vi "Car Wash.vi"() -> ()   [LabVIEW 2013]
doc: "This VI is a automated car wash simulation.\nIn initialize state all the controls will get enable and you have to select the control.\nOn pressing start, Car Warh Indicator start responding according to wash option.\n\nEach LED will glow for 5 sec.\nAfter then it will go to the next LED which is turned on from the wash option input\n\nIf the car position slider's position and wash option are not same then indicator will show Vehicle out of position.\n\nStop Program will stop the VI"
uses:
  Controls/Car Wash Indicators.ctl
  Controls/Wash Options.ctl
  Controls/States.ctl
  Controls/Wash option states.ctl
panel:
  in  "Start":bool
  out "Elapsed Time":dbl format="%0.2f"
  in  "stop":bool
  out "Wash Entry":bool
  in  "Wash Options":T1
  in  "Car Position Slider":u8(slide) max=3 scale=0.0..4.0
  out "Car Wash Indicators":T2
  # "Entry Console"
  # "Car Wash Display"
  # "Car Position Simulation"
  # "Pre-Soak\nH-P Wash\nL-P Wax\nSpot Free Rinse"
  # "Underbody Wash\nBug Remover"
  # "Tire Shine\nAir Dry"
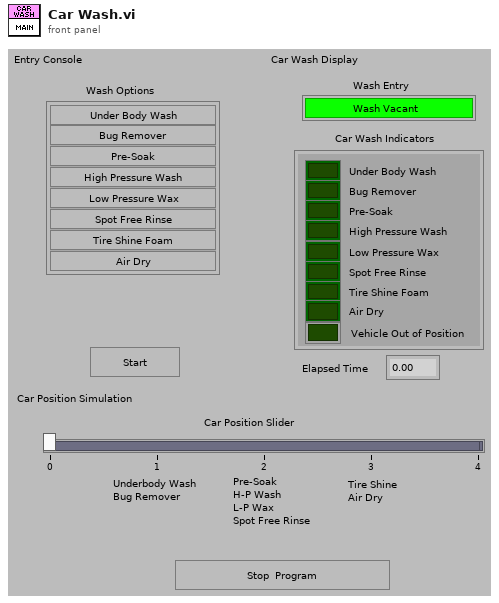
[diagram p1: front panel]
types:
  T1 = typedef "Wash Options.ctl" = cluster{"Underbody Wash":bool, "Bug Remover":bool, "Pre-Soak":bool, "High Pressure Wash":bool, "Low Pressure Wax":bool, "Spot Free Rinse":bool, "Tire Shine Foam":bool, "Air Dry":bool}
  T2 = typedef "Car Wash Indicators.ctl" = cluster{"Under Body Wash":bool, "Bug Remover":bool, "Pre-Soak":bool, "High Pressure Wash":bool, "Low Pressure Wax":bool, "Spot Free Rinse":bool, "Tire Shine Foam":bool, "Air Dry":bool, "Vehicle Out of Position":bool}
  T3 = typedef "Wash option states.ctl" = enum16{"Under Body Wash", "Bug Remover", "Pre-Soak", "HIgh Pressure Wash", "Low Pessure Wax", "Spot Free rinse", "Tire Shine Foam", "Air Dry", "Exit", "Reset "}
  T4 = typedef "States.ctl" = enum16{"Initialize", "Start", "Stop"}
  T5 = enum8{"Enabled", "Disabled", "Disabled and Grayed Out"}
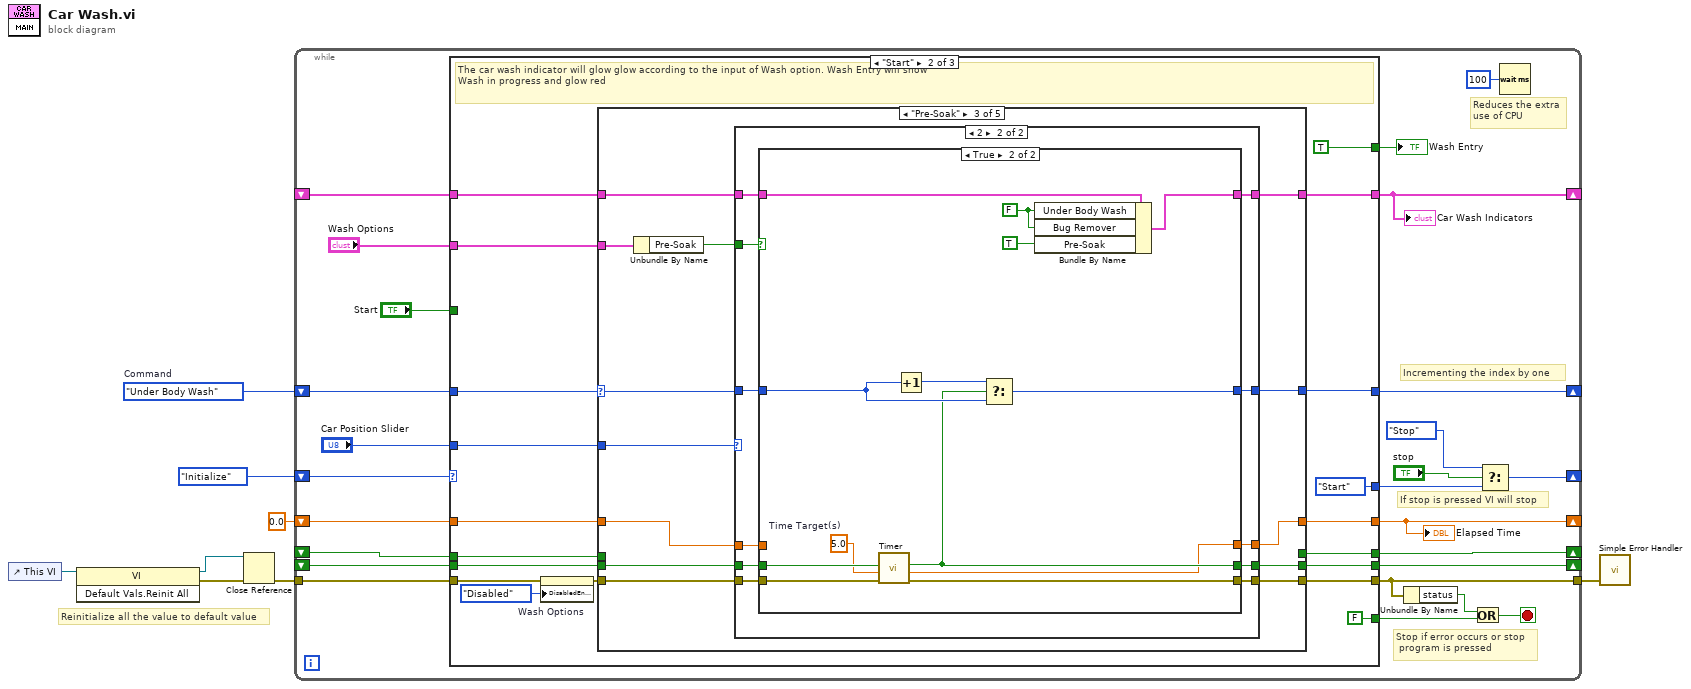
[diagram p0: block diagram]
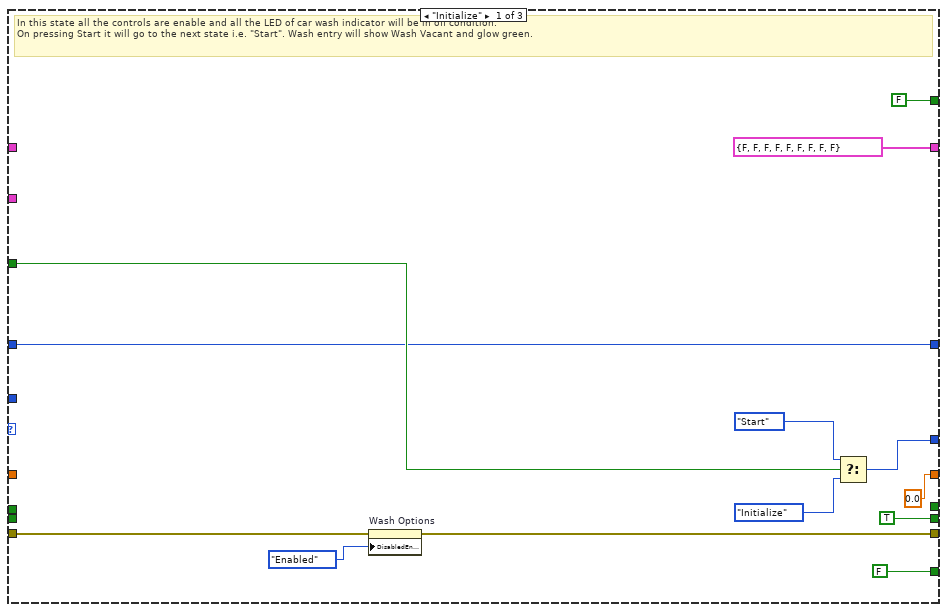
[diagram p2: hidden frame]
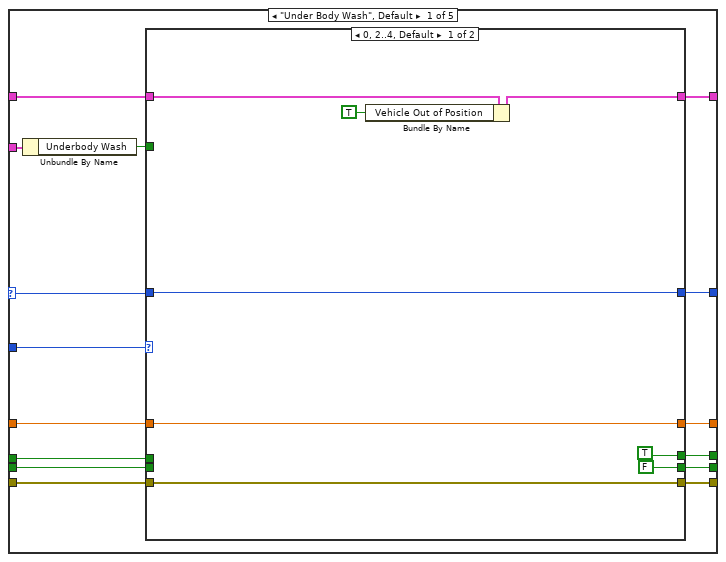
[diagram p3: hidden frame]
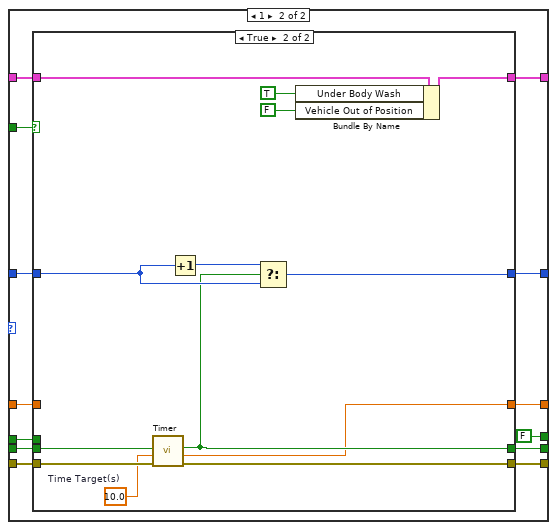
[diagram p4: hidden frame]
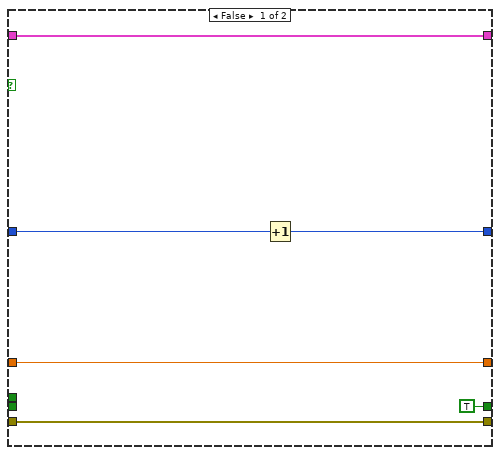
[diagram p5: hidden frame]
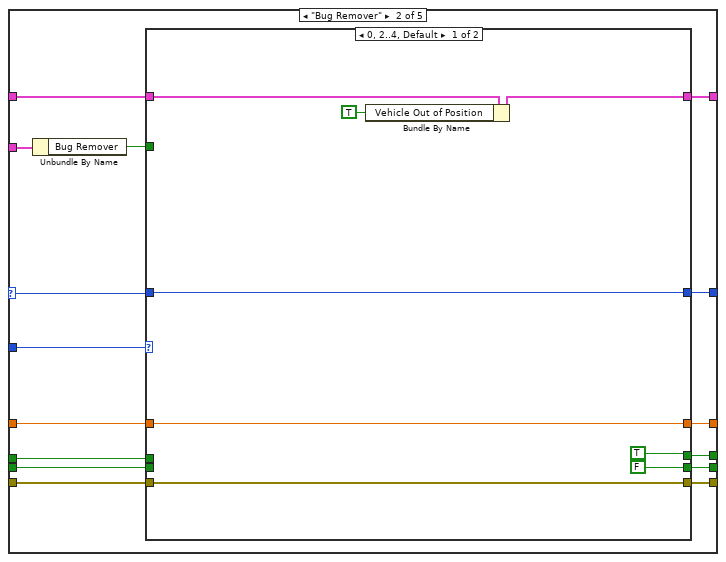
[diagram p6: hidden frame]
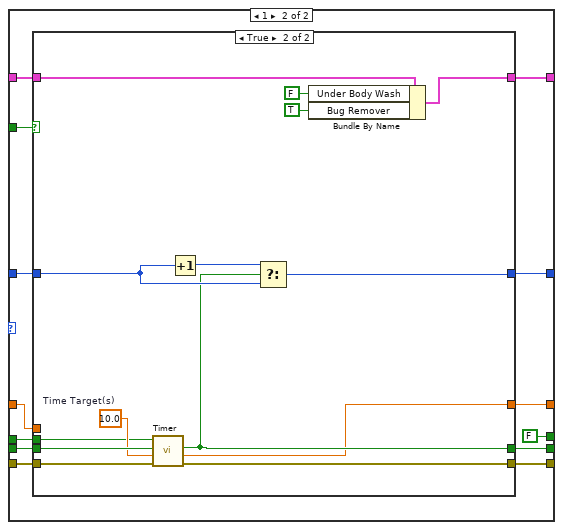
[diagram p7: hidden frame]
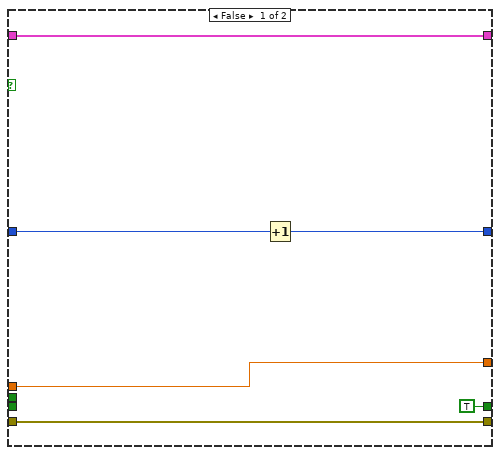
[diagram p8: hidden frame]
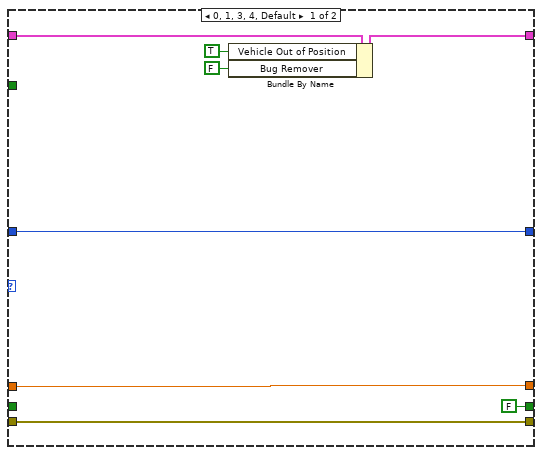
[diagram p9: hidden frame]
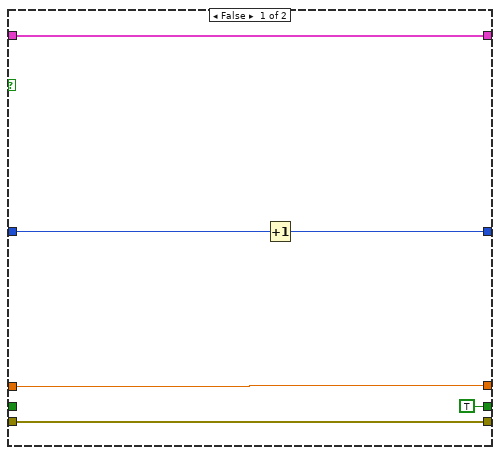
[diagram p10: hidden frame]
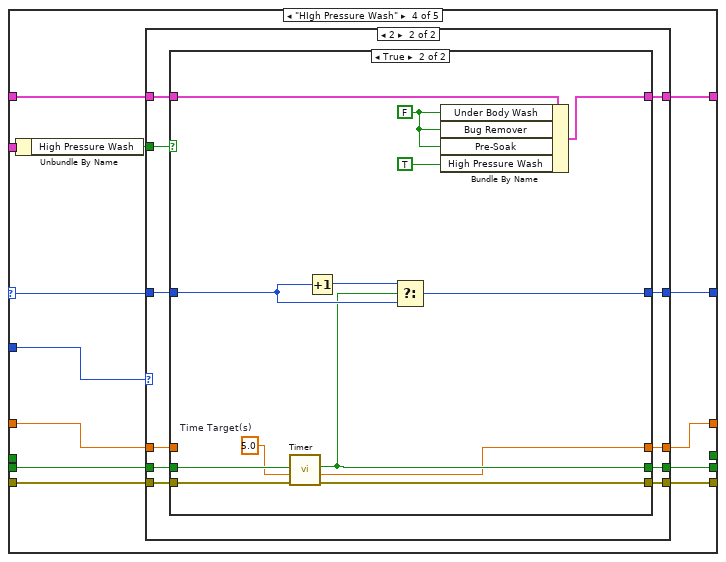
[diagram p11: hidden frame]
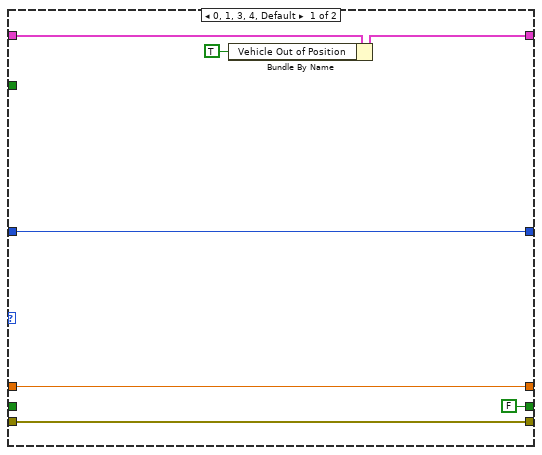
[diagram p12: hidden frame]
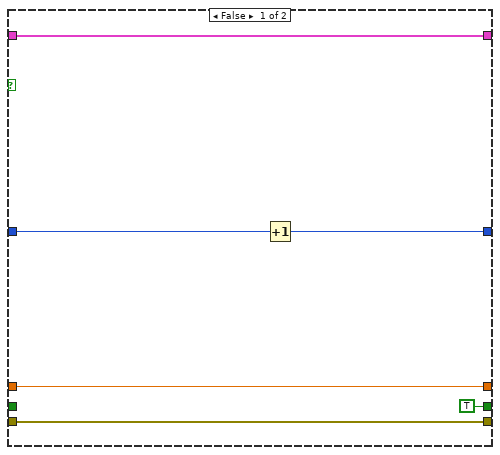
[diagram p13: hidden frame]
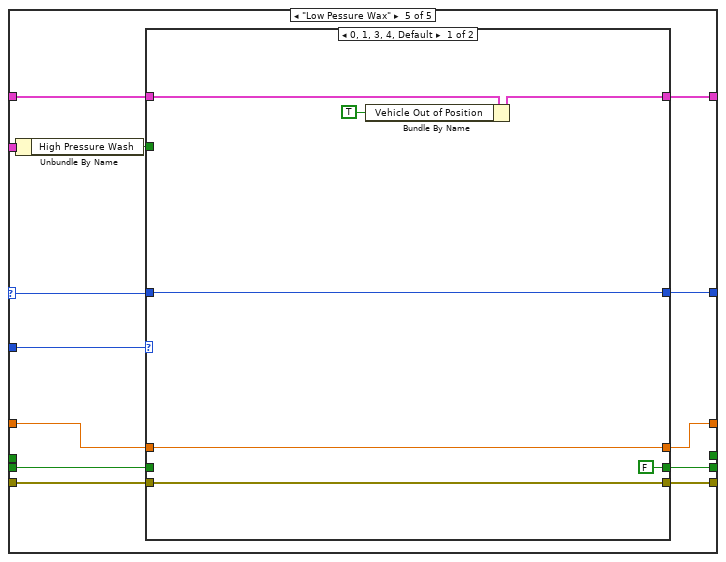
[diagram p14: hidden frame]
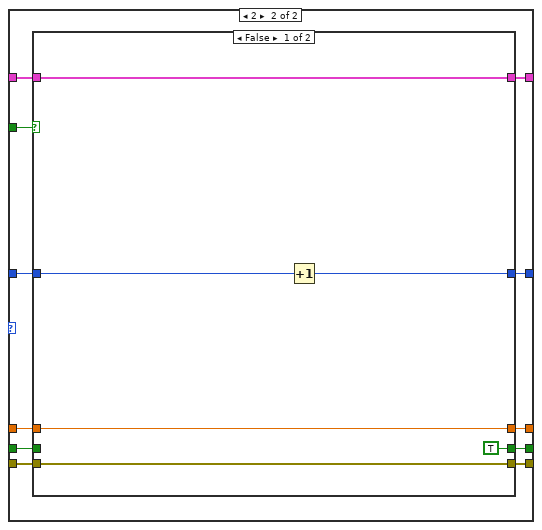
[diagram p15: hidden frame]
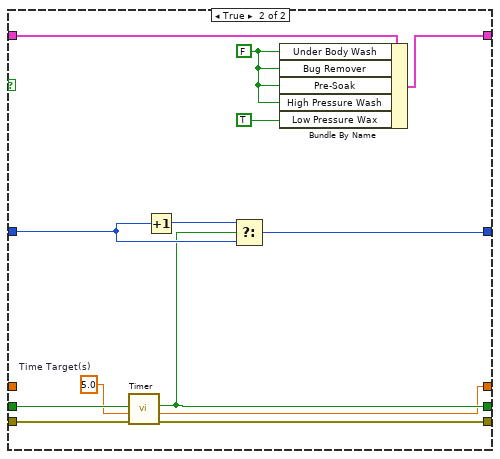
[diagram p16: hidden frame]
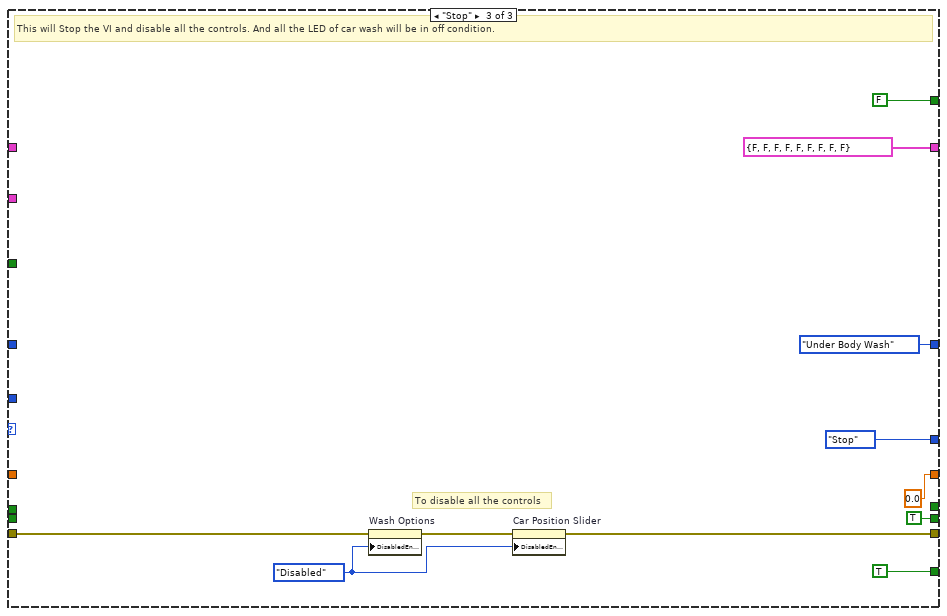
[diagram p17: hidden frame]
diagram:
  w2 = Wash_option_states."Under Body Wash"  # Command
  # "Reinitialize all the value to default value"
  n1 = control-ref of="This VI"() -> (w8:refnum<vi>)
  n2 = invoke class="VI" method="Default Vals.Reinit All"(reference=w8) -> (reference out=w6:refnum<vi>, error out=w7:errorcluster)  [unwired: 2 in, 1 out]
  n3 = Close Reference(reference=w6, error in (no error)=w7) -> (error out=w5:errorcluster)
  n4 = while {
    tunnel: w5 -> [w33]
    tunnel: [w32] -> w4
    shift-right: [w23] -> _
    shift-left: States."Initialize" -> [w28]
    shift-right: [w19] -> _
    shift-left: w2 -> [w20]
    shift-right: [w18] -> _
    shift-left: _ -> [w17]
    shift-right: [w15] -> _
    shift-left: _ -> [w14]
    shift-right: [w12] -> _
    shift-left: 0.0 ("Elapsed TIme") -> [w11]
    shift-right: [w9] -> _
    shift-left: _ -> [w10]
    stop <- w31 stop-if-true
    # "Incrementing the index by one"
    # "Reduces the extra\nuse of CPU"
    # "If stop is pressed VI will stop"
    # "Stop if error occurs or stop\n program is pressed"
    n5 = case shown="\"Start\"" w28 {
      tunnel: w33 -> [w44 w62 w336]
      tunnel: [w38 w56 w331] -> w32
      tunnel: [FALSE FALSE TRUE] -> w29
      tunnel: [FALSE TRUE FALSE] -> w27
      tunnel: [w41 States."Start" States."Stop"] -> w24
      tunnel: [T2 {"Under Body Wash"=FALSE, "Bug Remover"=FALSE, "Pre-Soak"=FALSE, "High Pressure Wash"=FALSE, "Low Pressure Wax"=FALSE, "Spot Free Rinse"=FALSE, "Tire Shine Foam"=FALSE, "Air Dry"=FALSE, "Vehicle Out of Position"=FALSE} ("Car Wash Indicators") w59 T2 {"Under Body Wash"=FALSE, "Bug Remover"=FALSE, "Pre-Soak"=FALSE, "High Pressure Wash"=FALSE, "Low Pressure Wax"=FALSE, "Spot Free Rinse"=FALSE, "Tire Shine Foam"=FALSE, "Air Dry"=FALSE, "Vehicle Out of Position"=FALSE} ("Car Wash Indicators")] -> w15
      tunnel: "Wash Options" -> [_ w52 _]
      tunnel: w20 -> [w35 w58 _]
      tunnel: [w35 w54 Wash_option_states."Under Body Wash" ("Command")] -> w19
      tunnel: [TRUE w51 TRUE] -> w18
      tunnel: w17 -> [_ w53 _]
      tunnel: "Start" -> [w36 _ _]
      tunnel: w14 -> [_ w60 _]
      tunnel: "Car Position Slider" -> [_ w55 _]
      tunnel: [0.0 ("Elapsed TIme") w50 0.0 ("Elapsed TIme")] -> w12
      tunnel: w11 -> [_ w49 _]
      tunnel: w10 -> [_ w48 _]
      tunnel: [_ w47 _] -> w9
      frame "Initialize" {
        # "In this state all the controls are enable and all the LED of car wash indicator will be in off condition.\nOn pressing Start it will go to the next state i.e. \"Start\". Wash entry will show Wash Vacant and glow green."
        n6 = property on="Wash Options" class="Clust (strict)"(error in=w44, "DisabledEnum"=T5."Enabled" ("Disabled")) -> (error out=w38:errorcluster)  [unwired: 1 in, 1 out]
        n7 = Select(t=States."Start", s=w36, f=States."Initialize") -> (s? t:f=w41:T4)
      }
      frame "Start" {
        # "The car wash indicator will glow glow according to the input of Wash option. Wash Entry will show \nWash in progress and glow red"
        n8 = property on="Wash Options" class="Clust (strict)"(error in=w62, "DisabledEnum"=T5."Disabled" ("Disabled")) -> (error out=w57:errorcluster)  [unwired: 1 in, 1 out]
        n9 = case shown="\"Pre-Soak\"" w58 {
          selector: w58 -> [w75 w130 w184 w235 w285]
          tunnel: w60 -> [w76 w131 w185 w236 w286]
          tunnel: [w77 w132 w186 w237 w287] -> w59
          tunnel: w57 -> [w80 w135 w189 w240 w290]
          tunnel: [w79 w134 w188 w239 w289] -> w56
          tunnel: w55 -> [w78 w133 w187 w238 w288]
          tunnel: [w74 w129 w183 w234 w284] -> w54
          tunnel: w53 -> [w73 w128 w182 w233 w283]
          tunnel: w52 -> [w72 w127 w181 w232 w282]
          tunnel: [w70 w125 w179 w230 w280] -> w51
          tunnel: [w69 w124 w178 w229 w279] -> w50
          tunnel: w49 -> [w68 w123 w177 w228 w278]
          tunnel: w48 -> [w67 w121 _ _ _]
          tunnel: [w66 w122 _ _ _] -> w47
          frame "Under Body Wash", Default {
            n10 = Unbundle By Name(w72) -> ("Underbody Wash"=w71:bool)
            n11 = case shown="0, 2..4, Default" w78 {
              tunnel: w80 -> [w83 w101]
              tunnel: [w83 w100] -> w79
              tunnel: [w87 w99] -> w77
              tunnel: w76 -> [w88 w98]
              tunnel: w75 -> [w85 w97]
              tunnel: [w85 w96] -> w74
              tunnel: w73 -> [_ w95]
              tunnel: w71 -> [_ w94]
              tunnel: [FALSE ("Elapsed?") w93] -> w70
              tunnel: [w81 w91] -> w69
              tunnel: w68 -> [w81 w92]
              tunnel: w67 -> [_ w90]
              tunnel: [TRUE ("Elapsed?") FALSE ("Elapsed?")] -> w66
              frame 0, 2..4, Default {
                n12 = Bundle By Name(cluster=w88, "Vehicle Out of Position"=TRUE) -> (w87:T2)
              }
              frame 1 {
                n13 = case shown="True" w94 {
                  tunnel: w101 -> [w104 w117]
                  tunnel: [w104 w116] -> w100
                  tunnel: [w106 w119] -> w99
                  tunnel: w98 -> [w106 w120]
                  tunnel: w97 -> [w107 w113]
                  tunnel: [w105 w114] -> w96
                  tunnel: w95 -> [_ w115]
                  tunnel: [TRUE ("Elapsed?") w111] -> w93
                  tunnel: w92 -> [w102 _]
                  tunnel: [w102 w109] -> w91
                  tunnel: w90 -> [_ _]
                  frame False {
                    n14 = Increment(x=w107) -> (x+1=w105:T3)
                  }
                  frame True {
                    w110 = 10.0  # Time Target(s)
                    n15 = call "Timer.vi"("error in (no error)"=w117, "Time Target(s)"=w110, "Reset"=w115) -> ("error out"=w116:errorcluster, "Elapsed TIme"=w109:dbl, "Elapsed?"=w111:bool)  [unwired: 6 in]
                    n16 = Increment(x=w113) -> (x+1=w112:T3)
                    n17 = Select(t=w112, s=w111, f=w113) -> (s? t:f=w114:T3)
                    n18 = Bundle By Name(cluster=w120, "Under Body Wash"=TRUE, "Vehicle Out of Position"=FALSE) -> (w119:T2)
                  }
                }
              }
            }
          }
          frame "Bug Remover" {
            n19 = Unbundle By Name(w127) -> ("Bug Remover"=w126:bool)
            n20 = case shown="0, 2..4, Default" w133 {
              tunnel: w135 -> [w138 w156]
              tunnel: [w138 w155] -> w134
              tunnel: [w142 w154] -> w132
              tunnel: w131 -> [w143 w153]
              tunnel: w130 -> [w140 w152]
              tunnel: [w140 w151] -> w129
              tunnel: w128 -> [_ w150]
              tunnel: w126 -> [_ w149]
              tunnel: [FALSE ("Elapsed?") w148] -> w125
              tunnel: [w137 w147] -> w124
              tunnel: w123 -> [w137 w146]
              tunnel: [TRUE ("Elapsed?") FALSE ("Elapsed?")] -> w122
              tunnel: w121 -> [_ w144]
              frame 0, 2..4, Default {
                n21 = Bundle By Name(cluster=w143, "Vehicle Out of Position"=TRUE) -> (w142:T2)
              }
              frame 1 {
                n22 = case shown="True" w149 {
                  tunnel: w156 -> [w159 w173]
                  tunnel: [w159 w172] -> w155
                  tunnel: [w161 w175] -> w154
                  tunnel: w153 -> [w161 w176]
                  tunnel: w152 -> [w162 w169]
                  tunnel: [w160 w170] -> w151
                  tunnel: w150 -> [_ w171]
                  tunnel: [TRUE ("Elapsed?") w167] -> w148
                  tunnel: [w157 w164] -> w147
                  tunnel: w146 -> [w157 _]
                  tunnel: w144 -> [_ w163]
                  frame False {
                    n23 = Increment(x=w162) -> (x+1=w160:T3)
                  }
                  frame True {
                    w166 = 10.0  # Time Target(s)
                    n24 = call "Timer.vi"("error in (no error)"=w173, "Time Target(s)"=w166, "Reset"=w171, "Pause"=w163) -> ("error out"=w172:errorcluster, "Elapsed TIme"=w164:dbl, "Elapsed?"=w167:bool)  [unwired: 5 in]
                    n25 = Increment(x=w169) -> (x+1=w168:T3)
                    n26 = Select(t=w168, s=w167, f=w169) -> (s? t:f=w170:T3)
                    n27 = Bundle By Name(cluster=w176, "Under Body Wash"=FALSE, "Bug Remover"=TRUE) -> (w175:T2)
                  }
                }
              }
            }
          }
          frame "Pre-Soak" {
            n28 = Unbundle By Name(w181) -> ("Pre-Soak"=w180:bool)
            n29 = case shown="2" w187 {
              tunnel: w189 -> [w192 w208]
              tunnel: [w192 w207] -> w188
              tunnel: [w196 w206] -> w186
              tunnel: w185 -> [w197 w205]
              tunnel: w184 -> [w194 w204]
              tunnel: [w194 w203] -> w183
              tunnel: w182 -> [_ w202]
              tunnel: w180 -> [_ w201]
              tunnel: [FALSE ("Elapsed?") w200] -> w179
              tunnel: [w190 w199] -> w178
              tunnel: w177 -> [w190 w198]
              frame 0, 1, 3, 4, Default {
                n30 = Bundle By Name(cluster=w197, "Vehicle Out of Position"=TRUE, "Bug Remover"=FALSE) -> (w196:T2)
              }
              frame 2 {
                n31 = case shown="True" w201 {
                  tunnel: w208 -> [w211 w225]
                  tunnel: [w211 w224] -> w207
                  tunnel: [w213 w226] -> w206
                  tunnel: w205 -> [w213 w227]
                  tunnel: w204 -> [w214 w221]
                  tunnel: [w212 w222] -> w203
                  tunnel: w202 -> [_ w223]
                  tunnel: [TRUE ("Elapsed?") w219] -> w200
                  tunnel: [w209 w215] -> w199
                  tunnel: w198 -> [w209 _]
                  frame False {
                    n32 = Increment(x=w214) -> (x+1=w212:T3)
                  }
                  frame True {
                    w218 = 5.0  # Time Target(s)
                    w216 = FALSE ("Under Body Wash")
                    n33 = call "Timer.vi"("error in (no error)"=w225, "Time Target(s)"=w218, "Reset"=w223) -> ("error out"=w224:errorcluster, "Elapsed TIme"=w215:dbl, "Elapsed?"=w219:bool)  [unwired: 6 in]
                    n34 = Increment(x=w221) -> (x+1=w220:T3)
                    n35 = Select(t=w220, s=w219, f=w221) -> (s? t:f=w222:T3)
                    n36 = Bundle By Name(cluster=w227, "Under Body Wash"=w216, "Bug Remover"=w216, "Pre-Soak"=TRUE ("Bug Remover")) -> (w226:T2)
                  }
                }
              }
            }
          }
          frame "HIgh Pressure Wash" {
            n37 = Unbundle By Name(w232) -> ("High Pressure Wash"=w231:bool)
            n38 = case shown="2" w238 {
              tunnel: w240 -> [w242 w258]
              tunnel: [w242 w257] -> w239
              tunnel: [w246 w256] -> w237
              tunnel: w236 -> [w247 w255]
              tunnel: w235 -> [w244 w254]
              tunnel: [w244 w253] -> w234
              tunnel: w233 -> [_ w252]
              tunnel: w231 -> [_ w251]
              tunnel: [FALSE ("Elapsed?") w250] -> w230
              tunnel: [w241 w249] -> w229
              tunnel: w228 -> [w241 w248]
              frame 0, 1, 3, 4, Default {
                n39 = Bundle By Name(cluster=w247, "Vehicle Out of Position"=TRUE) -> (w246:T2)
              }
              frame 2 {
                n40 = case shown="True" w251 {
                  tunnel: w258 -> [w261 w275]
                  tunnel: [w261 w274] -> w257
                  tunnel: [w263 w276] -> w256
                  tunnel: w255 -> [w263 w277]
                  tunnel: w254 -> [w264 w271]
                  tunnel: [w262 w272] -> w253
                  tunnel: w252 -> [_ w273]
                  tunnel: [TRUE ("Elapsed?") w269] -> w250
                  tunnel: [w259 w265] -> w249
                  tunnel: w248 -> [w259 _]
                  frame False {
                    n41 = Increment(x=w264) -> (x+1=w262:T3)
                  }
                  frame True {
                    w268 = 5.0  # Time Target(s)
                    w266 = FALSE ("Under Body Wash")
                    n42 = call "Timer.vi"("error in (no error)"=w275, "Time Target(s)"=w268, "Reset"=w273) -> ("error out"=w274:errorcluster, "Elapsed TIme"=w265:dbl, "Elapsed?"=w269:bool)  [unwired: 6 in]
                    n43 = Increment(x=w271) -> (x+1=w270:T3)
                    n44 = Select(t=w270, s=w269, f=w271) -> (s? t:f=w272:T3)
                    n45 = Bundle By Name(cluster=w277, "Under Body Wash"=w266, "Bug Remover"=w266, "Pre-Soak"=w266, "High Pressure Wash"=TRUE ("Bug Remover")) -> (w276:T2)
                  }
                }
              }
            }
          }
          frame "Low Pessure Wax" {
            n46 = Unbundle By Name(w282) -> ("High Pressure Wash"=w281:bool)
            n47 = case shown="0, 1, 3, 4, Default" w288 {
              tunnel: w290 -> [w292 w308]
              tunnel: [w292 w307] -> w289
              tunnel: [w296 w306] -> w287
              tunnel: w286 -> [w297 w305]
              tunnel: w285 -> [w294 w304]
              tunnel: [w294 w303] -> w284
              tunnel: w283 -> [_ w302]
              tunnel: w281 -> [_ w301]
              tunnel: [FALSE ("Elapsed?") w300] -> w280
              tunnel: [w291 w299] -> w279
              tunnel: w278 -> [w291 w298]
              frame 0, 1, 3, 4, Default {
                n48 = Bundle By Name(cluster=w297, "Vehicle Out of Position"=TRUE) -> (w296:T2)
              }
              frame 2 {
                n49 = case shown="False" w301 {
                  tunnel: w308 -> [w311 w325]
                  tunnel: [w311 w324] -> w307
                  tunnel: [w313 w326] -> w306
                  tunnel: w305 -> [w313 w327]
                  tunnel: w304 -> [w314 w321]
                  tunnel: [w312 w322] -> w303
                  tunnel: w302 -> [_ w323]
                  tunnel: [TRUE ("Elapsed?") w319] -> w300
                  tunnel: [w309 w315] -> w299
                  tunnel: w298 -> [w309 _]
                  frame False {
                    n50 = Increment(x=w314) -> (x+1=w312:T3)
                  }
                  frame True {
                    w318 = 5.0  # Time Target(s)
                    w316 = FALSE ("Under Body Wash")
                    n51 = call "Timer.vi"("error in (no error)"=w325, "Time Target(s)"=w318, "Reset"=w323) -> ("error out"=w324:errorcluster, "Elapsed TIme"=w315:dbl, "Elapsed?"=w319:bool)  [unwired: 6 in]
                    n52 = Increment(x=w321) -> (x+1=w320:T3)
                    n53 = Select(t=w320, s=w319, f=w321) -> (s? t:f=w322:T3)
                    n54 = Bundle By Name(cluster=w327, "Under Body Wash"=w316, "Bug Remover"=w316, "Pre-Soak"=w316, "High Pressure Wash"=w316, "Low Pressure Wax"=TRUE ("Bug Remover")) -> (w326:T2)
                  }
                }
              }
            }
          }
        }
      }
      frame "Stop" {
        w330 = T5."Disabled" ("Disabled")
        # "To disable all the controls"
        # "This will Stop the VI and disable all the controls. And all the LED of car wash will be in off condition."
        n55 = property on="Wash Options" class="Clust (strict)"(error in=w336, "DisabledEnum"=w330) -> (error out=w332:errorcluster)  [unwired: 1 in, 1 out]
        n56 = property on="Car Position Slider" class="Slide (strict)"(error in=w332, "DisabledEnum"=w330) -> (error out=w331:errorcluster)  [unwired: 1 in, 1 out]
      }
    }
    "Wash Entry" <- w27
    "Car Wash Indicators" <- w15
    "Elapsed Time" <- w12
    n57 = Unbundle By Name(w32) -> ("status"=w30:bool)
    n58 = Or(x=w30, y=w29) -> (x .or. y?=w31:bool)
    n59 = Select(t=States."Stop", s="stop", f=w24) -> (s? t:f=w23:T4)
    n60 = Wait (ms)(milliseconds to wait=u32 100) -> ()  [unwired: 1 out]
  }
  n61 = call <vilib>:"Simple Error Handler.vi"("error in (no error)"=w4) -> ()  [unwired: 4 in, 5 out]
